vi "Load_Position_Limit.vi"(0 "Serial In":refnum<visa-resource-name>, 5 "Node":u8, 7 "Upper Limit":i64, 9 "Lower Limit":i64, 11 "Error In":errorcluster) -> (4 "Serial Out":refnum<visa-resource-name>, 15 "Error Out":errorcluster)   [LabVIEW 2019, in "Faulhaber RS232.lvlib"]
uses:
  <instrlib>/Faulhaber RS232/Faulhaber RS232.lvlib
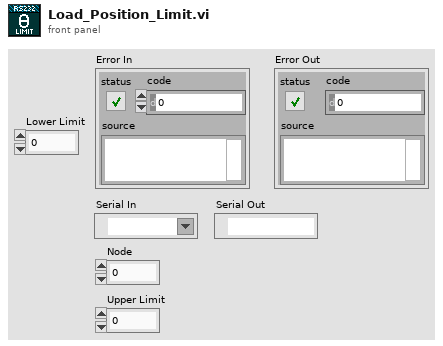
[diagram p1: front panel]
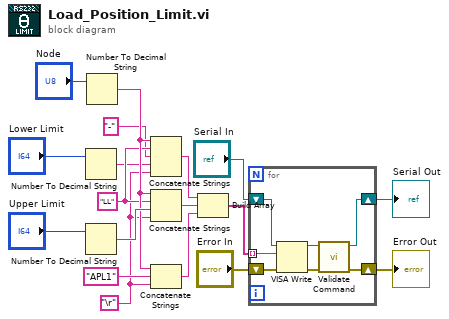
[diagram p0: block diagram]
diagram:
  w10 = "LL" ("string")
  w4 = "\r"
  n1 = Number To Decimal String(number="Lower Limit") -> (decimal integer string=w5:string)  [unwired: 1 in]
  n2 = Number To Decimal String(number="Upper Limit") -> (decimal integer string=w12:string)  [unwired: 1 in]
  n3 = Number To Decimal String(number="Node") -> (decimal integer string=w11:string)  [unwired: 1 in]
  n4 = Concatenate Strings(w11, w10, "-" ("string"), w5, w4) -> (w1:string)
  n5 = Concatenate Strings(w11, w10, w12, w4) -> (w2:string)
  n6 = Concatenate Strings(w11, "APL1" ("string"), w4) -> (w8:string)
  n7 = Build Array(w1, w2, w8) -> (w7:string[])
  n8 = for {
    tunnel: w7 -> [w23] mode=indexing
    shift-right: [w21] -> w15
    shift-left: "Serial In" -> [w25]
    shift-right: [w19] -> w16
    shift-left: "Error In" -> [w24]
    n9 = VISA Write(VISA resource name=w25, write buffer=w23, error in (no error)=w24) -> (VISA resource name out=w22:refnum<visa-resource-name>, error out=w20:errorcluster)  [unwired: 1 out]
    n10 = call <instrlib>:"Validate Command.vi"("error in (no error)"=w20, "Serial in"=w22) -> ("error out"=w19:errorcluster, "Serial Out"=w21:refnum<visa-resource-name>)  [unwired: 3 in, 1 out]
  }
  "Error Out" <- w16
  "Serial Out" <- w15
